vi "SR430.get address.vi"(0 "i ref in":refnum<vi>, 5 "error in (no error)":errorcluster) -> (14 "i ref out":refnum<vi>, 16 "address":T1, 19 "error out":errorcluster)   [LabVIEW 2014, in "SR430.lvlib"]
doc: "gets the GPIB address out of the BaseProcess i attributes. That string is needed when calling the instrument driver within the methods of this class."
uses:
  SR430.lvlib
  CSinstr.lib/Sr430/SR430_VISA Control.ctl
  CSCore/BaseProcess/BaseProcess.lvlib
  CSinstr.lib/Sr430/SR430Driver.lvlib
panel:
  in  "SR430 VISA type":T1
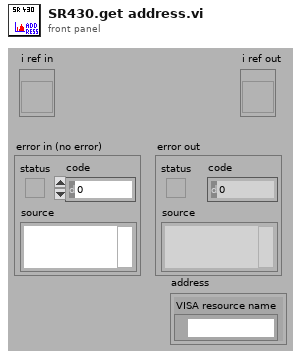
[diagram p1: front panel]
types:
  T1 = typedef "SR430Driver.lvlib/SR430_VISA Control.ctl" = cluster{"VISA resource name":refnum<visa-resource-name>}
  T2 = typedef "BaseProcess.lvlib/BaseProcess.i attribute.ctl" = cluster{"EventStatus":string, "EventError":i32, "PresetEvtWatchD":i32, "PresetPdcWatchD":i32, "EventTimeout":i32, "PeriodicInterval":i32, "Interface":string[], "Address":string[], "Special":string[], "PeriodicError":i32, "PeriodicStatus":string, "SuperProc":string, "Descriptors":T3[], "CaseRef":refnum<vi>, "PdcRef":refnum<vi>, "Thread Ref":refnum<vi>, "eventErrorID":i32, "eventStatusID":i32, "periodicErrorID":i32, "periodicStatusID":i32, "pdcCtrID":i32}
  T3 = typedef "BaseProcess.lvlib/BaseProcess.descriptor definition.ctl" = cluster{"selector":string, "descriptor":T4}
  T4 = typedef "BaseProcess.lvlib/BaseProcess.descriptor string definition.ctl" = string
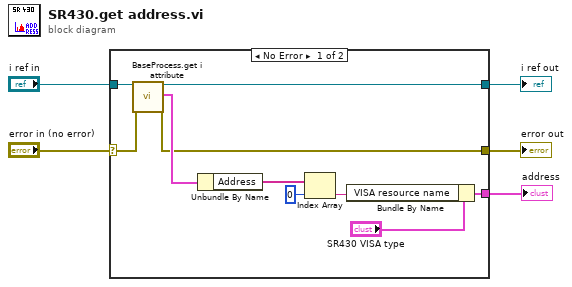
[diagram p0: block diagram]
diagram:
  n1 = case shown="No Error" "error in (no error)" {
    selector: "error in (no error)" -> [w9 w16]
    tunnel: "i ref in" -> [w15 w17]
    tunnel: [w6 _] -> w4
    tunnel: [w11 w17] -> w3
    tunnel: [w10 w16] -> w2
    frame No Error {
      n2 = call "BaseProcess.get i attribute.vi"("i ref in"=w15, "error in (no error)"=w9) -> ("i ref out"=w11:refnum<vi>, "i attribute"=w12:T2, "error out"=w10:errorcluster)  [unwired: 15 in]
      n3 = Unbundle By Name(w12) -> ("Address"=w13:string[])
      n4 = Index Array(array=w13, index=0 ("Index")) -> (element=w7:string)
      n5 = Bundle By Name(cluster="SR430 VISA type", "VISA resource name"=w7) -> (w6:T1)
    }
    frame Error {
    }
  }
  "error out" <- w2
  "i ref out" <- w3
  "address" <- w4
